vi "Demodulate symbols.vi"(0 "input complex waveform":T1={"t0"=0.0, "dt"=1.0, "Y"=[]} {"Y" format="%.3f"; "dt" format="%^.2e"; "t0" format="%.4f"}, 5 "PSK system parameters":T2={"samples per symbol (16)"=16, "symbol map"=[]} {"symbol map" format="%.3f"}, 7 "matched filter coefficients":dbl[](array[numeric]) format="%.2f", 9 "Number of Symbols":i32, 11 "error in (no error)":errorcluster, 12 "TX Pulse Shaping Filter Coefficients":dbl[](array[numeric]) format="%.2f") -> (4 "Output Bit Stream":i8[](array[numeric]), 6 "output complex waveform":T1={"t0"=0.0, "dt"=1.0, "Y"=[]} {"Y" format="%.3f"; "dt" format="%^.2e"; "t0" format="%.4f"}, 15 "error out":errorcluster)   [LabVIEW 2011]
uses:
  <vilib>/addons/Modulation/Analog/controls/Complex Data Waveform.ctl
  <vilib>/addons/Modulation/niAMT.lvlib
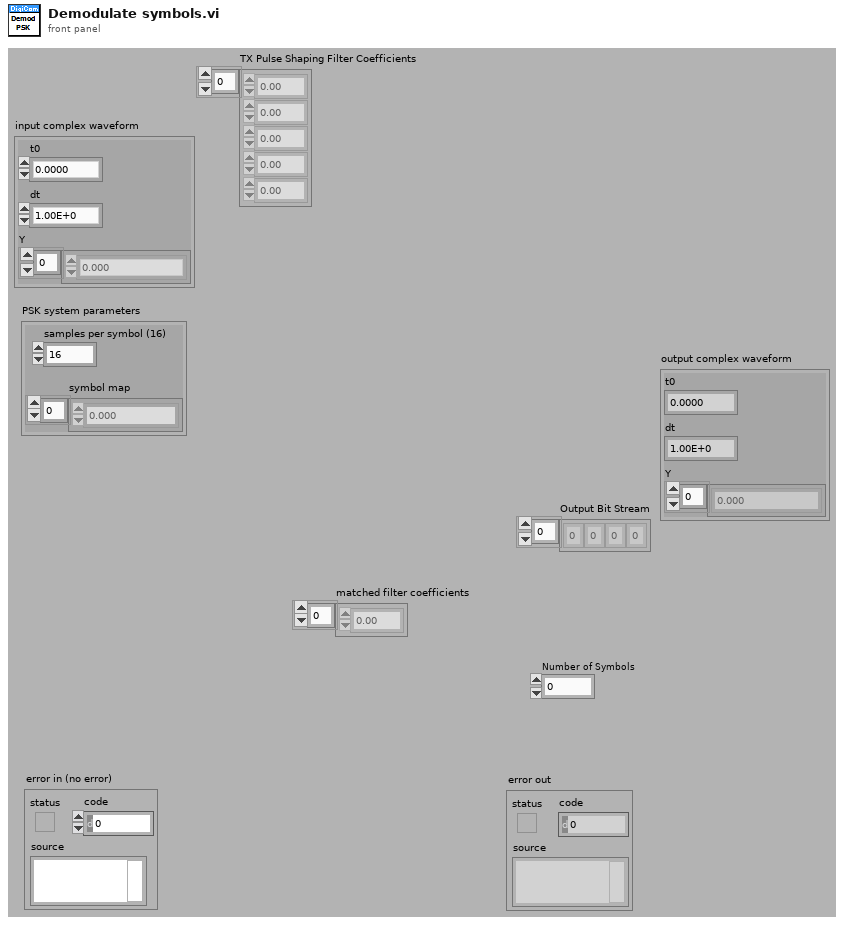
[diagram p1: front panel]
types:
  T1 = typedef "niAMT.lvlib/Complex Data Waveform.ctl" = cluster{"t0":dbl, "dt":dbl, "Y":cdb[]}
  T2 = cluster{"samples per symbol (16)":i32, "symbol map":cdb[]}
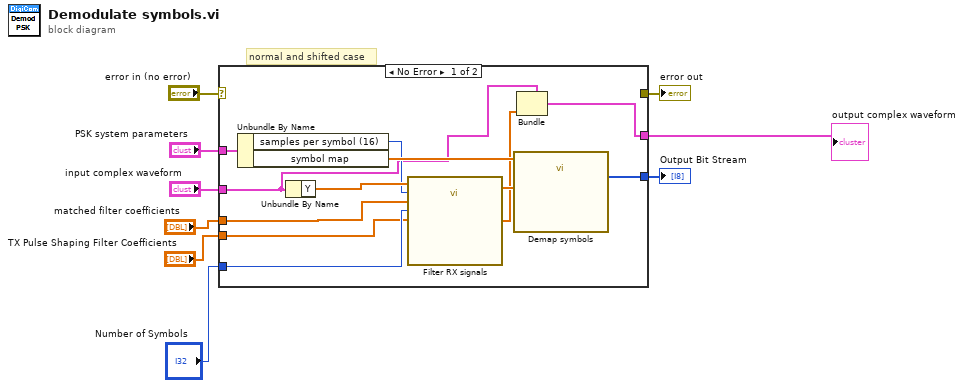
[diagram p0: block diagram]
diagram:
  # "normal and shifted case"
  n1 = case shown="No Error" "error in (no error)" {
    selector: "error in (no error)" -> [_ w22]
    tunnel: "input complex waveform" -> [w14 _]
    tunnel: [_ w22] -> w7
    tunnel: "matched filter coefficients" -> [w11 _]
    tunnel: "PSK system parameters" -> [w20 _]
    tunnel: [w18 _] -> w4
    tunnel: "Number of Symbols" -> [w15 _]
    tunnel: [w12 _] -> w2
    tunnel: "TX Pulse Shaping Filter Coefficients" -> [w10 _]
    frame No Error {
      n2 = Unbundle By Name(w20) -> ("samples per symbol (16)"=w16:i32, "symbol map"=w19:cdb[])
      n3 = Unbundle By Name(w14) -> ("Y"=w17:cdb[])
      n4 = call "Filter RX signals.vi"("Symbols"=w17, "Samples Per Symbol (16)"=w16, "RX Matched Filter Coefficients"=w11, "Number of Symbols"=w15, "TX Pulse Shaping Filter Coefficients"=w10) -> ("decimated symbols"=w21:cdb[], "Filtered Samples"=w13:cdb[])  [unwired: 4 in]
      n5 = call "Demap symbols.vi"("Symbols"=w21, "Symbol Map"=w19) -> ("Output Bit Stream"=w18:i8[])  [unwired: 7 in]
      n6 = Bundle(cluster=w14, "Y"=w13) -> (w12:T1)  [unwired: 2 in]
    }
    frame Error {
    }
  }
  "error out" <- w7
  "Output Bit Stream" <- w4
  "output complex waveform" <- w2
